vi "PH_PPMA_PowerUnit.ProcEvents.vi"(0 "i ref in":refnum<vi>, 5 "error in (no error)":errorcluster) -> (14 "i ref out":refnum<vi>, 19 "error out":errorcluster)   [LabVIEW 2014, in "PH_PPMA_PowerUnit.lvlib"]
doc: "This method is used to define the events the object will listen to. Add your own events here."
uses:
  PH_PPMA_PowerUnit.lvlib
  CSCore/BaseProcess/BaseProcess.event definition.ctl
  CSCore/CAEObj/CAEObj.event definition.ctl
  CSCore/BaseProcess/BaseProcess.descriptor string definition.ctl
  PH_PP_Common/PH_PP_Common.Trigger Tags.ctl
  PH_PP_Common/PH_PP_Common.PSU Tags.ctl
  PH_Beckhoff_PP_PU/PH_Beckhoff_PP_PU.Igni Tags.ctl
  PH_Beckhoff_PP_PU/PH_Beckhoff_PP_PU.RR Tags.ctl
  PH_Beckhoff_PP_Control/PH_Beckhoff_PP_Control.PP Mercury Tags.ctl
  PH_Beckhoff_PPMA-Rods/PH_Beckhoff_PPMA-Rods.Rods Tags.ctl
  CSCore/BaseProcess/BaseProcess.lvlib
  CSCore/CAEObj/CAEObj.lvlib
  PH_Common/PH_Common.lvlib
  PH_Beckhoff_PP_Control/PH_Beckhoff_PP_Control.lvlib
  PH_Beckhoff_PPMA-Rods/PH_Beckhoff_PPMA-Rods.lvlib
  PH_PP_Common/PH_PP_Common.lvlib
  PH_Beckhoff_PP_PU/PH_Beckhoff_PP_PU.lvlib
  PH_PowerUnit_BaseClass/PH_PowerUnit_BaseClass.lvlib
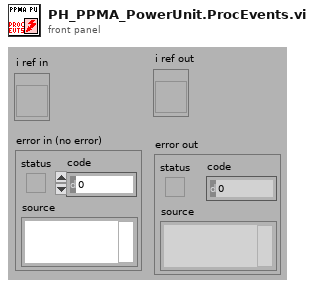
[diagram p1: front panel]
types:
  T1 = typedef "PH_Beckhoff_PP_Control.lvlib/PH_Beckhoff_PP_Control.PP Mercury Tags.ctl" = enum16{"Device-on", "Alarm", "on-since", "Concentration", "Status"}
  T2 = typedef "PH_Beckhoff_PP_PU.lvlib/PH_Beckhoff_PP_PU.RR Tags.ctl" = enum16{"open", "closed", "close", "Status"}
  T3 = typedef "PH_Beckhoff_PP_PU.lvlib/PH_Beckhoff_PP_PU.Igni Tags.ctl" = enum16{"heating-on", "water-on", "Device-on", "Status"}
  T4 = typedef "BaseProcess.lvlib/BaseProcess.event definition.ctl" = cluster{"CAEEvtDef":T5, "Data Descriptor":T6}
  T5 = typedef "CAEObj.lvlib/CAEObj.event definition.ctl" = cluster{"URL":string, "enable":bool, "ignoreResID":bool}
  T6 = typedef "BaseProcess.lvlib/BaseProcess.descriptor string definition.ctl" = string
  T7 = typedef "PH_Beckhoff_PPMA-Rods.lvlib/PH_Beckhoff_PPMA-Rods.Rods Tags.ctl" = enum16{"Rod-up", "earth-ok", "door-locked-K1", "door-locked-K2", "watervalve-closed", "Rods-Chain-A-up", "Rods-Chain-B-up", "HV-Warnlamp-orange", "HV-Warnlamp-green", "Status-Rods-PU-1", "Status-Rods-PU-2", "Status-Rods-PU-3", "Status-Rods-PU-4", "Status-Rods-PU-5", "Status-Rods-PU-6", "Status-Rods-PU-7", "Status-Rods-PU-8", "Status-Rods-PU-9", "Status-Rods-PU-10", "Status-Rods-FR", "Status-Rods-PILC"}
  T8 = typedef "PH_PP_Common.lvlib/PH_PP_Common.PSU Tags.ctl" = enum16{"voltage-indicator", "peak-detect", "current", "voltage", "inihibit-indicator", "end-of-charge", "HV-on-indicator", "overtemperature", "interlock-indicator", "load-fault", "sum-fault", "HV-off-indicator", "DC-ok", "inhibit", "HV-on", "interlock", "reset", "Status", "Limits"}
  T9 = typedef "PH_PP_Common.lvlib/PH_PP_Common.Trigger Tags.ctl" = enum16{"triggered", "fired", "Status", "Last Shot"}
  T10 = typedef "PH_PowerUnit_BaseClass.lvlib/PH_PowerUnit_BaseClass.i attribute.ctl" = cluster{"Constructor finished":bool, "PU":cluster{"In use":bool, "Service ID in use":i32, "GUI Ref":refnum<vi>}, "Enabling":cluster{"State":T11, "GUI Ref":refnum<vi>}, "Timing":cluster{"Last Shot":dbl, "Time between Shots [Sec]":dbl, "Waiting Time over?":bool, "Service ID Waiting Time":i32, "GUI Ref":refnum<vi>, "Instance":cluster{"Status":T12, "linked?":bool, "GUI Ref":refnum<vi>}}, "Sequencer":cluster{"SM State":string, "GUI Ref":refnum<vi>, "linked":bool}, "Subscribed Trendmssgs":cluster{"Tagname":string, "Status":T12, "linked?":bool, "Shot Condition":T12, "GUI Ref":refnum<vi>}[], "PP PU":T13, "Default Voltage (V)":dbl, "GUI Refs":T14, "PSDB data":cluster{"Shot Voltage [V]":dbl, "State TO SM":T15, "Write 2 early":bool}, "State TO SM":T15}
  T11 = typedef "PH_SystemInformation.lvlib/PH_SystemInformationEnabling State.ctl" = i32
  T12 = typedef "PH_StatusHandler.lvlib/PH_StatusHandler.Status.ctl" = i16
  T13 = typedef "PH_PP_Common.lvlib/PH_PP_Common.PUs.ctl" = enum16{"no Info", "PA-19mm-1", "PA-19mm-2", "PA-45mm-PILC", "PA-45mm-MAIN", "MA-PU-1", "MA-PU-2", "MA-PU-3", "MA-PU-4", "MA-PU-5", "MA-PU-6", "MA-FR", "MA-PILC", "PA-45mm-DP"}
  T14 = typedef "PH_PowerUnit_BaseClass.lvlib/PH_PowerUnit_BaseClass.GUI Refs.ctl" = cluster{"Delete Inst":refnum<vi>, "State TO SM":refnum<vi>, "State SM":refnum<vi>, "Fire":refnum<vi>}
  T15 = typedef "PH_PowerUnit_BaseClass.lvlib/PH_PowerUnit_BaseClass.SM States.ctl" = enum16{".", "Stand by", "Switch PU on", "Configure", "Set Default Voltage", "Set STANDBY", "Set READY", "Wait for Shot Cmd", "Open Dump Rods", "Open Ross Relais", "Close Ross Relais", "Switch PSU on", "Switch PSU off", "Charge", "Switch GD Channel on", "Close Dump Rods", "Rods-TO", "RR-TO", "PSU-TO", "Trigger-TO"}
  T16 = typedef "PH_Common.lvlib/PH_DIM.Event Declarer.ctl" = cluster{"Service Name":string, "Selector":string}
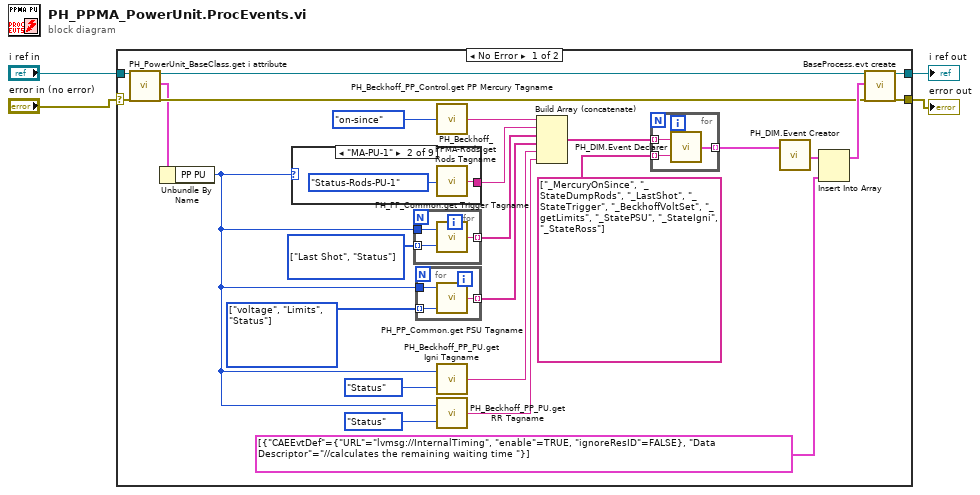
[diagram p0: block diagram]
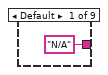
[diagram p2: hidden frame]
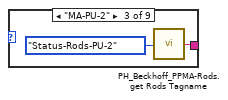
[diagram p3: hidden frame]
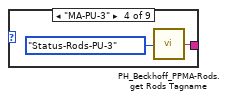
[diagram p4: hidden frame]
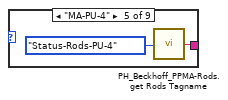
[diagram p5: hidden frame]
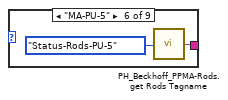
[diagram p6: hidden frame]
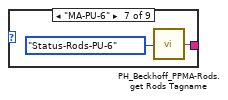
[diagram p7: hidden frame]
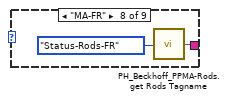
[diagram p8: hidden frame]
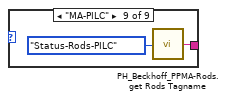
[diagram p9: hidden frame]
diagram:
  n1 = case shown="No Error" "error in (no error)" {
    selector: "error in (no error)" -> [w8 w56]
    tunnel: [w28 w57] -> w4
    tunnel: [w27 w56] -> w3
    tunnel: "i ref in" -> [w9 w57]
    frame No Error {
      w15 = T8[] [enum."voltage", enum."Limits", enum."Status"] items=["voltage-indicator", "peak-detect", "current", "voltage", "inihibit-indicator", "end-of-charge", "HV-on-indicator", "overtemperature", "interlock-indicator", "load-fault", "sum-fault", "HV-off-indicator", "DC-ok", "inhibit", "HV-on", "interlock", "reset", "Status", "Limits"]
      w17 = T9[] [enum."Last Shot", enum."Status"] items=["triggered", "fired", "Status", "Last Shot"]
      n2 = call "PH_PowerUnit_BaseClass.get i attribute.vi"("i ref in"=w9, "error in (no error)"=w8) -> ("i ref out"=w23:refnum<vi>, "i attribute"=w6:T10, "error out"=w22:errorcluster)  [unwired: 15 in]
      n3 = Unbundle By Name(w6) -> ("PP PU"=w5:T13)
      n4 = case shown="\"MA-PU-1\"" w5 {
        tunnel: ["N/A" ("Rods Tagname") w37 w39 w41 w43 w45 w47 w49 w51] -> w18
        frame Default {
        }
        frame "MA-PU-1" {
          n5 = call "PH_Beckhoff_PPMA-Rods.get Rods Tagname.vi"("Rods Tag"=PH_Beckhoff_PPMA-Rods.Rods_Tags."Status-Rods-PU-1") -> ("Rods Tagname"=w37:string)
        }
        frame "MA-PU-2" {
          n6 = call "PH_Beckhoff_PPMA-Rods.get Rods Tagname.vi"("Rods Tag"=PH_Beckhoff_PPMA-Rods.Rods_Tags."Status-Rods-PU-2") -> ("Rods Tagname"=w39:string)
        }
        frame "MA-PU-3" {
          n7 = call "PH_Beckhoff_PPMA-Rods.get Rods Tagname.vi"("Rods Tag"=PH_Beckhoff_PPMA-Rods.Rods_Tags."Status-Rods-PU-3") -> ("Rods Tagname"=w41:string)
        }
        frame "MA-PU-4" {
          n8 = call "PH_Beckhoff_PPMA-Rods.get Rods Tagname.vi"("Rods Tag"=PH_Beckhoff_PPMA-Rods.Rods_Tags."Status-Rods-PU-4") -> ("Rods Tagname"=w43:string)
        }
        frame "MA-PU-5" {
          n9 = call "PH_Beckhoff_PPMA-Rods.get Rods Tagname.vi"("Rods Tag"=PH_Beckhoff_PPMA-Rods.Rods_Tags."Status-Rods-PU-5") -> ("Rods Tagname"=w45:string)
        }
        frame "MA-PU-6" {
          n10 = call "PH_Beckhoff_PPMA-Rods.get Rods Tagname.vi"("Rods Tag"=PH_Beckhoff_PPMA-Rods.Rods_Tags."Status-Rods-PU-6") -> ("Rods Tagname"=w47:string)
        }
        frame "MA-FR" {
          n11 = call "PH_Beckhoff_PPMA-Rods.get Rods Tagname.vi"("Rods Tag"=PH_Beckhoff_PPMA-Rods.Rods_Tags."Status-Rods-FR") -> ("Rods Tagname"=w49:string)
        }
        frame "MA-PILC" {
          n12 = call "PH_Beckhoff_PPMA-Rods.get Rods Tagname.vi"("Rods Tag"=PH_Beckhoff_PPMA-Rods.Rods_Tags."Status-Rods-PILC") -> ("Rods Tagname"=w51:string)
        }
      }
      n13 = for {
        tunnel: w5 -> [w35]
        tunnel: w17 -> [w34] mode=indexing
        tunnel: [w33] -> w16 mode=indexing
        n14 = call "PH_PP_Common.get Trigger Tagname.vi"("Trigger Tag"=w34, "PU"=w35) -> ("Trigger Tagname"=w33:string)
      }
      n15 = for {
        tunnel: w5 -> [w32]
        tunnel: w15 -> [w31] mode=indexing
        tunnel: [w30] -> w14 mode=indexing
        n16 = call "PH_PP_Common.get PSU Tagname.vi"("PSU Tag"=w31, "PU"=w32) -> ("PSU Tagname"=w30:string)  [unwired: 1 in]
      }
      n17 = call "PH_Beckhoff_PP_Control.get PP Mercury Tagname.vi"("PP Mercury Tag"=PH_Beckhoff_PP_Control.PP_Mercury_Tags."on-since") -> ("PP Mercury Tagname"=w19:string)
      n18 = call "PH_Beckhoff_PP_PU.get Igni Tagname.vi"("Igni Tag"=PH_Beckhoff_PP_PU.Igni_Tags."Status", "PU"=w5) -> ("Igni Tagname"=w12:string)
      n19 = call "PH_Beckhoff_PP_PU.get RR Tagname.vi"("Ross Relais Tag"=PH_Beckhoff_PP_PU.RR_Tags."Status", "PU"=w5) -> ("RR Tagname"=w10:string)
      n20 = Build Array (concatenate)(w19, w18, w16, w14, w12, w10) -> (w21:string[])
      n21 = for {
        tunnel: w21 -> [w54] mode=indexing
        tunnel: string[] ["_MercuryOnSince", "_StateDumpRods", "_LastShot", "_StateTrigger", "_BeckhoffVoltSet", "_getLimits", "_StatePSU", "_StateIgni", "_StateRoss"] -> [w53] mode=indexing
        tunnel: [w55] -> w26 mode=indexing
        n22 = call "PH_DIM.Event Declarer.vi"("Selector"=w53, "Service Name"=w54) -> ("declared DIM Event"=w55:T16)
      }
      n23 = call "PH_DIM.Event Creator.vi"("Trendmessage Services"=w26) -> ("DIM Service Events"=w25:T4[])  [unwired: 18 in]
      n24 = Insert Into Array(array=w25, new element=T4[] [{"CAEEvtDef"={"URL"="lvmsg://InternalTiming", "enable"=TRUE, "ignoreResID"=FALSE}, "Data Descriptor"="//calculates the remaining waiting time "}] ("new events")) -> (w29:T4[])  [unwired: 1 in]
      n25 = call "BaseProcess.evt create.vi"("i ref in"=w23, "newEvents"=w29, "error in (no error)"=w22) -> ("i ref out"=w28:refnum<vi>, "error out"=w27:errorcluster)  [unwired: 13 in, 2 out]
    }
    frame Error {
    }
  }
  "i ref out" <- w4
  "error out" <- w3
